vi "Gain to Coarse Gain Index.vi"(0 "gain setting":fxp<+/-,16,12>, 5 "coarse gain values":fxp<+/-,16,12>[](array[numeric])=[0.0, 0.0, 0.0, 0.0]) -> (4 "coarse gain index":u32)   [LabVIEW 2019]
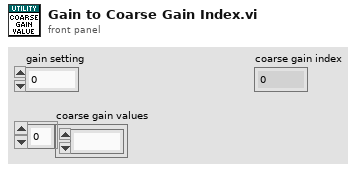
[diagram p1: front panel]
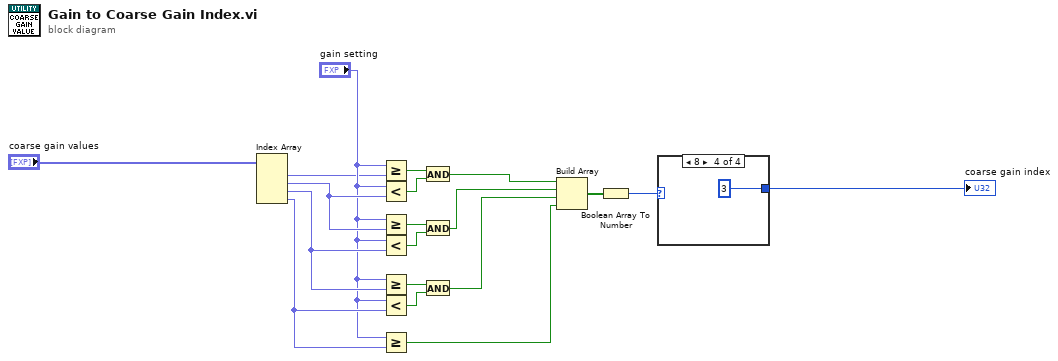
[diagram p0: block diagram]
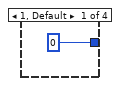
[diagram p2: hidden frame]
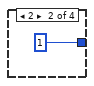
[diagram p3: hidden frame]
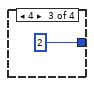
[diagram p4: hidden frame]
diagram:
  n1 = Index Array(array="coarse gain values") -> (element #1=w8:fxp<+/-,16,12>, element #2=w14:fxp<+/-,16,12>, element #3=w15:fxp<+/-,16,12>, element #4=w16:fxp<+/-,16,12>)  [unwired: 4 in]
  n2 = Greater Or Equal?(x="gain setting", y=w8) -> (x >= y?=w1:bool)
  n3 = Less?(x="gain setting", y=w14) -> (x < y?=w2:bool)
  n4 = Greater Or Equal?(x="gain setting", y=w14) -> (x >= y?=w10:bool)
  n5 = Less?(x="gain setting", y=w15) -> (x < y?=w9:bool)
  n6 = Greater Or Equal?(x="gain setting", y=w15) -> (x >= y?=w11:bool)
  n7 = Less?(x="gain setting", y=w16) -> (x < y?=w12:bool)
  n8 = Greater Or Equal?(x="gain setting", y=w16) -> (x >= y?=w19:bool)
  n9 = And(x=w1, y=w2) -> (x .and. y?=w3:bool)
  n10 = And(x=w10, y=w9) -> (x .and. y?=w17:bool)
  n11 = And(x=w11, y=w12) -> (x .and. y?=w18:bool)
  n12 = Build Array(w3, w17, w18, w19) -> (w4:bool[])
  n13 = Boolean Array To Number(Boolean array=w4) -> (number=w5:u8)
  n14 = case shown="8" w5 {
    tunnel: [u32 0 ("fast jump table index") u32 1 ("fast jump table index") u32 2 ("fast jump table index") u32 3 ("fast jump table index")] -> w6
    frame 1, Default {
    }
    frame 2 {
    }
    frame 4 {
    }
    frame 8 {
    }
  }
  "coarse gain index" <- w6
